vi "Untitled 1 (SubVI).vi"(6 "cam 0":T1, 7 "S arrays":T2, 9 "CamSettings":T3, 10 "Clibration":T7={"cam 0"={"incident ANGLE COMPENSATION"=[], "field of view /pixel"=0.0, "dp/B [MeV/C/B]"=[], "charge compensation"=[], "Momentum [MeV/C]"=[], "B [T]"=0.0, "energyDependence Input"=[], "pixel angle (y)"=[], "dp [MeV/C/] "=[], "angle 2Dfor spectrumj"=[], "dp [MeV/C] 2D"=[], "charge compensation 2D"=[], "Screen&Cam"={"Screen Orientation"="", "Screen angle"="", "Lens"="", "Calibration (mm/pix)"=0.0}, "ROI info"={"npix-X"=0, "npix-Y"=0, "Left [pix]"=0.0, "Top [pix]"=0.0}}, "cam 1"={"incident ANGLE COMPENSATION"=[], "field of view /pixel"=0.0, "dp/B [MeV/C/B]"=[], "charge compensation"=[], "Momentum [MeV/C]"=[], "B [T]"=1.0, "energyDependence Input"=[], "pixel angle (y)"=[], "dp [MeV/C/] "=[], "angle 2Dfor spectrumj"=[], "dp [MeV/C] 2D"=[], "charge compensation 2D"=[], "Screen&Cam"={"Screen Orientation"="", "Screen angle"="", "Lens"="", "Calibration (mm/pix)"=0.0}, "ROI info"={"npix-X"=0, "npix-Y"=0, "Left [pix]"=0.0, "Top [pix]"=0.0}}, "cam 2"={"incident ANGLE COMPENSATION"=[], "field of view /pixel"=0.0, "dp/B [MeV/C/B]"=[], "charge compensation"=[], "Momentum [MeV/C]"=[], "B [T]"=1.0, "energyDependence Input"=[], "pixel angle (y)"=[], "dp [MeV/C/] "=[], "angle 2Dfor spectrumj"=[], "dp [MeV/C] 2D"=[], "charge compensation 2D"=[], "Screen&Cam"={"Screen Orientation"="", "Screen angle"="", "Lens"="", "Calibration (mm/pix)"=0.0}, "ROI info"={"npix-X"=0, "npix-Y"=0, "Left [pix]"=0.0, "Top [pix]"=0.0}}, "cam 3"={"incident ANGLE COMPENSATION"=[], "field of view /pixel"=0.0, "dp/B [MeV/C/B]"=[], "charge compensation"=[], "Momentum [MeV/C]"=[], "B [T]"=1.0, "energyDependence Input"=[], "pixel angle (y)"=[], "dp [MeV/C/] "=[], "angle 2Dfor spectrumj"=[], "dp [MeV/C] 2D"=[], "charge compensation 2D"=[], "Screen&Cam"={"Screen Orientation"="", "Screen angle"="", "Lens"="", "Calibration (mm/pix)"=0.0}, "ROI info"={"npix-X"=0, "npix-Y"=0, "Left [pix]"=0.0, "Top [pix]"=0.0}}}, 11 "Refnum in":T1) -> (1 "Cam Cluster out 2":T8={"incident ANGLE COMPENSATION"=[], "field of view /pixel"=0.0, "dp/B [MeV/C/B]"=[], "charge compensation"=[], "Momentum [MeV/C]"=[], "B [T]"=1.0, "energyDependence Input"=[], "pixel angle (y)"=[], "dp [MeV/C/] "=[], "angle 2Dfor spectrumj"=[], "dp [MeV/C] 2D"=[], "charge compensation 2D"=[], "Screen&Cam"={"Screen Orientation"="", "Screen angle"="", "Lens"="", "Calibration (mm/pix)"=0.0}, "ROI info"={"npix-X"=0, "npix-Y"=0, "Left [pix]"=0.0, "Top [pix]"=0.0}}, 2 "spec cluster":cluster{"dp [MeV/C]":dbl[], dbl[]}(graph), 3 "z":dbl[][](graph), 4 "Cam Cluster out 3":T8)   [LabVIEW 2011]
uses:
  calib_Sub_Typdef.ctl
  ScreenCam_TypDEf.ctl
  ROIInfo_TypDef.ctl
  Calib_Typdef.ctl
  CamSettings_Typdef.ctl
  CamSettingSUB_TypDEf.ctl
  lens_TypDEf.ctl
  shared/OnOffTypeDef.ctl
  <vilib>/vision/Image Controls.llb/IMAQ Image.ctl
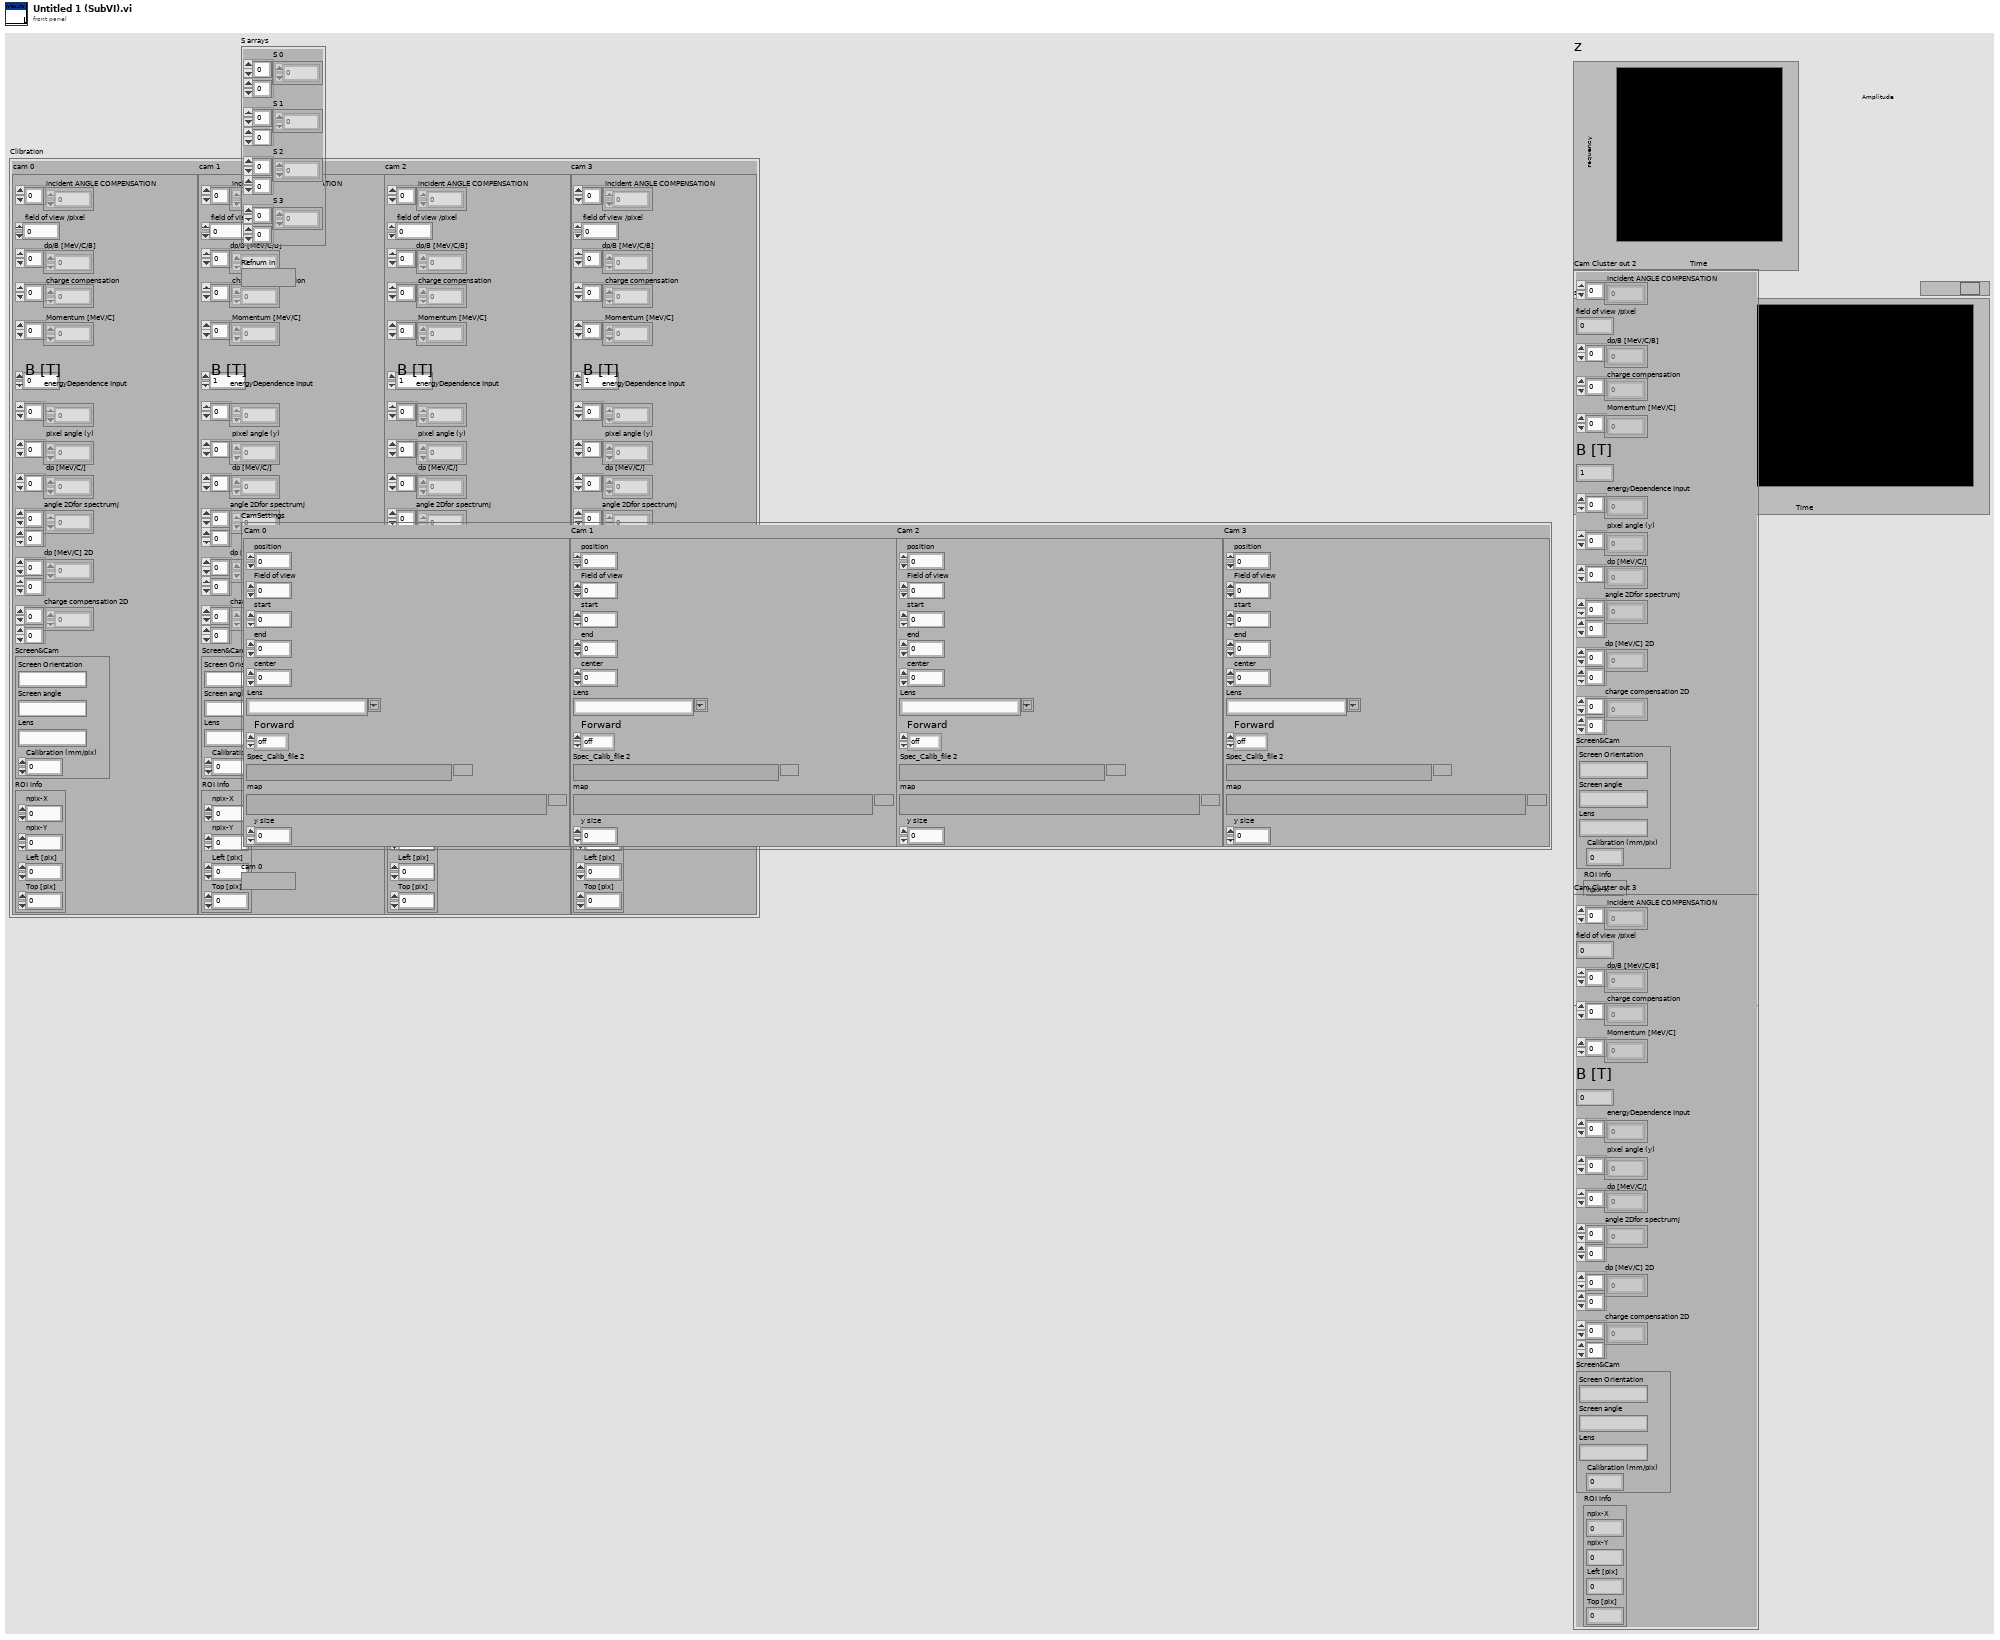
[diagram p1: front panel]
types:
  T1 = typedef "IMAQ Image.ctl" = refnum<image>
  T2 = cluster{"S 0":i32[][], "S 1":i32[][], "S 2":i32[][], "S 3":i32[][]}
  T3 = typedef "CamSettings_Typdef.ctl" = cluster{"Cam 0":T4, "Cam 1":T4, "Cam 2":T4, "Cam 3":T4}
  T4 = typedef "CamSettingSUB_TypDEf.ctl" = cluster{"position":dbl, "Field of view":dbl, "start":dbl, "end":dbl, "center":dbl, "Lens":T5, "Forward":T6, "Spec_Calib_file 2":path, "map":path, "y size":i32}
  T5 = typedef "lens_TypDEf.ctl" = string
  T6 = typedef "OnOffTypeDef.ctl" = enum16{"off", "on"}
  T7 = typedef "Calib_Typdef.ctl" = cluster{"cam 0":T8, "cam 1":T8, "cam 2":T8, "cam 3":T8}
  T8 = typedef "calib_Sub_Typdef.ctl" = cluster{"incident ANGLE COMPENSATION":dbl[], "field of view /pixel":dbl, "dp/B [MeV/C/B]":dbl[], "charge compensation":dbl[], "Momentum [MeV/C]":dbl[], "B [T]":dbl, "energyDependence Input":dbl[], "pixel angle (y)":dbl[], "dp [MeV/C/] ":dbl[], "angle 2Dfor spectrumj":dbl[][], "dp [MeV/C] 2D":dbl[][], "charge compensation 2D":dbl[][], "Screen&Cam":T9, "ROI info":T10}
  T9 = typedef "ScreenCam_TypDEf.ctl" = cluster{"Screen Orientation":string, "Screen angle":string, "Lens":string, "Calibration (mm/pix)":dbl}
  T10 = typedef "ROIInfo_TypDef.ctl" = cluster{"npix-X":i32, "npix-Y":i32, "Left [pix]":dbl, "Top [pix]":dbl}
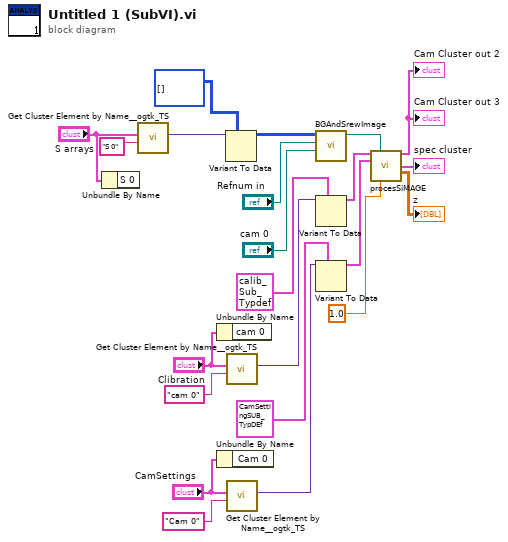
[diagram p0: block diagram]
diagram:
  n1 = Unbundle By Name("S arrays") -> ()  [unwired: 1 out]
  n2 = call "Get Cluster Element by Name__ogtk_TS.vi"("Element Name"="S 0", "Cluster"="S arrays") -> ("VElement"=w9:variant)  [unwired: 7 in, 2 out]
  n3 = Unbundle By Name("Clibration") -> ()  [unwired: 1 out]
  n4 = Unbundle By Name("CamSettings") -> ()  [unwired: 1 out]
  n5 = Variant To Data(type=i32[][] [] ("S 0"), Variant=w9) -> (data=w11:i32[][])  [unwired: 1 in, 1 out]
  n6 = call "Get Cluster Element by Name__ogtk_TS.vi"("Element Name"="cam 0", "Cluster"="Clibration") -> ("VElement"=w19:variant)  [unwired: 7 in, 2 out]
  n7 = call "Get Cluster Element by Name__ogtk_TS.vi"("Element Name"="Cam 0", "Cluster"="CamSettings") -> ("VElement"=w12:variant)  [unwired: 7 in, 2 out]
  n8 = call "BGAndSrewImage.vi"("BG Image"="cam 0", "Image"="Refnum in", "S arrays.S 0"=w11) -> ("Image Out"=w1:T1)  [unwired: 6 in, 2 out]
  n9 = Variant To Data(type=T8 {"incident ANGLE COMPENSATION"=[], "field of view /pixel"=0.0, "dp/B [MeV/C/B]"=[], "charge compensation"=[], "Momentum [MeV/C]"=[], "B [T]"=1.0, "energyDependence Input"=[], "pixel angle (y)"=[], "dp [MeV/C/] "=[], "angle 2Dfor spectrumj"=[], "dp [MeV/C] 2D"=[], "charge compensation 2D"=[], "Screen&Cam"={"Screen Orientation"="", "Screen angle"="", "Lens"="", "Calibration (mm/pix)"=0.0}, "ROI info"={"npix-X"=0, "npix-Y"=0, "Left [pix]"=0.0, "Top [pix]"=0.0}} ("cam 0"), Variant=w19) -> (data=w21:T8)  [unwired: 1 in, 1 out]
  n10 = Variant To Data(type=T4 {"position"=0.0, "Field of view"=0.0, "start"=0.0, "end"=0.0, "center"=0.0, "Lens"="f8x06", "Forward"=enum."off", "Spec_Calib_file 2"=path "Y:/100TWdata/ESMCalib/datFwd.txt", "map"=path "Y:/100TWdata/ESMCalib/mapFwd.txt", "y size"=0} ("Cam 0"), Variant=w12) -> (data=w16:T4)  [unwired: 1 in, 1 out]
  n11 = call "procesSiMAGE.vi"("Cam Cluster out"=w21, "Image"=w1, "CamSettings.Cam 0"=w16, "B [T]"=1.0) -> ("Cam Cluster out 2"=→"Cam Cluster out 2" →"Cam Cluster out 3":T8, "spec cluster"=→"spec cluster":cluster{"dp [MeV/C]":dbl[], dbl[]}, "z"=→"z":dbl[][])  [unwired: 8 in, 1 out]
